vi "Create PAS Data.vi"(8 "error in (no error)":errorcluster) -> (0 "error out":errorcluster, 3 "CreatePASData":refnum<k24>)   [LabVIEW 2015]
uses:
  C:/Distributed/CalFlex.dll
  CalFlex.dll
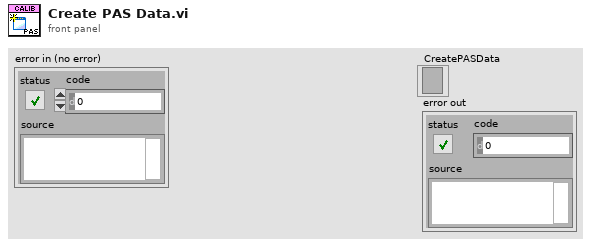
[diagram p1: front panel]
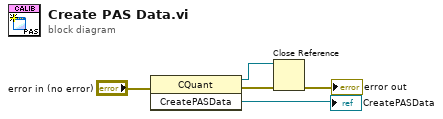
[diagram p0: block diagram]
diagram:
  n1 = invoke class="CQuant" method="CreatePASData"(error in="error in (no error)") -> (reference out=w4:refnum<k24>, error out=w5:errorcluster, "CreatePASData"=→"CreatePASData":refnum<k24>)  [unwired: 2 in]
  n2 = Close Reference(reference=w4, error in (no error)=w5) -> (error out=→"error out":errorcluster)
